vi "Check If Environment Variable Exists.vi"(7 "Target (Process)":T1 items=["Process", "User", "Machine"], 8 "Error In":errorcluster, 11 "Name":string) -> (0 "Error Out":errorcluster, 3 "Exists?":bool)   [LabVIEW 2019, in "SLL Environment Variable.lvlib"]
doc: "Check if the environment variable exists in the target environment."
uses:
  <vilib>/SLL Toolkit/SLL Environment Variable/SLL Environment Variable.lvlib
  <vilib>/SLL Toolkit/SLL Environment Variable/_Typedef/Target Environment Enum.ctl
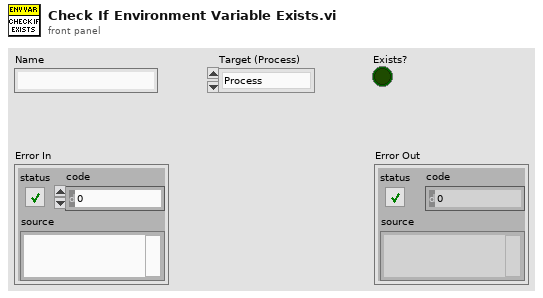
[diagram p1: front panel]
types:
  T1 = typedef "SLL Environment Variable.lvlib/Target Environment Enum.ctl" = i32
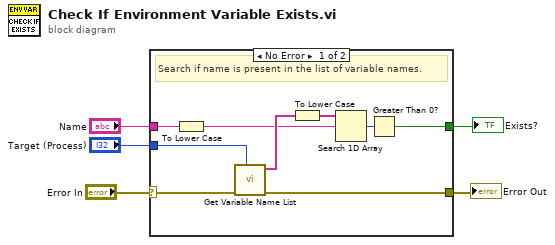
[diagram p0: block diagram]
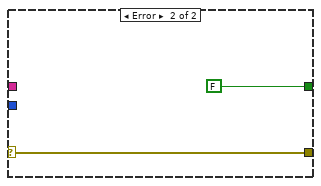
[diagram p2: hidden frame]
diagram:
  n1 = case shown="No Error" "Error In" {
    selector: "Error In" -> [w6 w15]
    tunnel: [w14 w15] -> w5
    tunnel: "Target (Process)" -> [w13 _]
    tunnel: "Name" -> [w11 _]
    tunnel: [w7 FALSE] -> w2
    frame No Error {
      # "Search if name is present in the list of variable names."
      n2 = To Lower Case(string=w11) -> (all lower case string=w10:string)
      n3 = call <vilib>:"Get Variable Name List.vi"("Target (Process)"=w13, "Error In"=w6) -> ("Error Out"=w14:errorcluster, "Names[]"=w12:string[])  [unwired: 8 in]
      n4 = To Lower Case(string=w12) -> (all lower case string=w9:string[])
      n5 = Search 1D Array(1D array=w9, element=w10) -> (index of element=w8:i32)  [unwired: 1 in]
      n6 = Greater Than 0?(x=w8) -> (x > 0?=w7:bool)
    }
    frame Error {
    }
  }
  "Error Out" <- w5
  "Exists?" <- w2
